vi "Tidal Eng-Write Temperature Setpoint.vi"(6 "Temperature Setpoint":T1=40100 items=["Ch1 Setpoint"=40100, "Ch1 Process Variable"=40103, "Ch2 Setpoint"=40200, "Ch2 Process Variable"=40203, "Ch3 Setpoint"=40300, "Ch3 Process Variable"=40303, "All Events Mask"=40500, "Run State"=40600], 8 "error in (no error)":errorcluster, 10 "Temperature (°F)":dbl=1.0, 11 "Modbus master in":refnum<class "Modbus Master.lvclass">) -> (0 "error out":errorcluster, 3 "Modbus master out":refnum<class "Modbus Master.lvclass">)   [LabVIEW 2023]
uses:
  Type Definitions/Tenney Modbus Registers.ctl
  <vilib>/NI/Modbus Library/API/Master/Modbus Master.lvclass
panel:
  out "unsigned Setpoint":u16
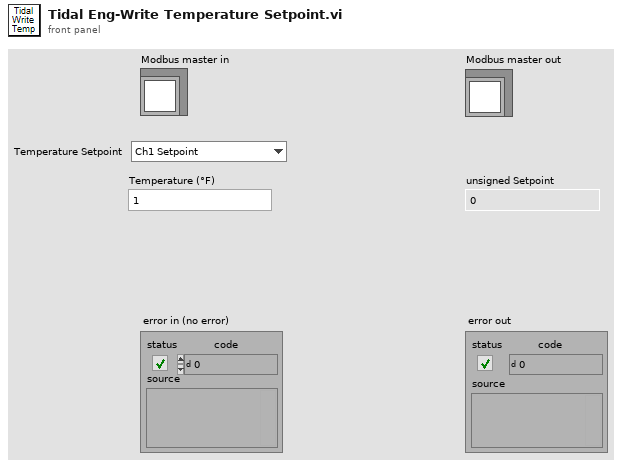
[diagram p1: front panel]
types:
  T1 = typedef "Tenney Modbus Registers.ctl" = u16
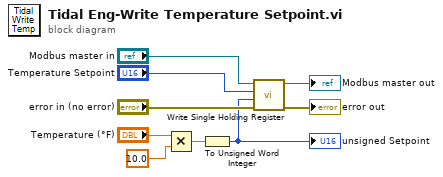
[diagram p0: block diagram]
diagram:
  n1 = Multiply(x="Temperature (°F)", y=10.0) -> (x*y=w2:dbl)
  n2 = To Unsigned Word Integer(number=w2) -> (unsigned 16bit integer=w1:u16)
  "unsigned Setpoint" <- w1
  n3 = call-dynamic "Write Single Holding Register.vi"("error in"="error in (no error)", "register to write"=w1, "address"="Temperature Setpoint", "Modbus master in"="Modbus master in") -> ("error out"=→"error out":errorcluster, "Modbus master out"=→"Modbus master out":refnum<class "Modbus Master.lvclass">)  [unwired: 6 in]
